vi "histograma.vi"(0 "Array":T1(array[cluster])) -> (14 "XY Graph 2":T1(graph))   [LabVIEW 2019]
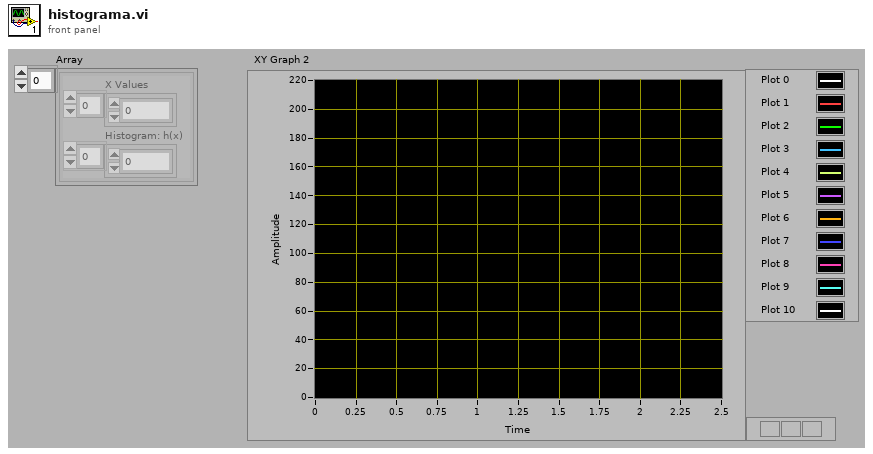
[diagram p1: front panel]
types:
  T1 = cluster{"X Values":dbl[], "Histogram: h(x)":i32[]}[]
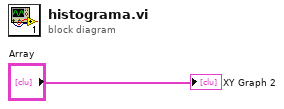
[diagram p0: block diagram]
diagram:
  "XY Graph 2" <- "Array"
